vi "Relink Subroutine Test Exec.vi"(4 "Path Builder":refnum<class "IPath Builder.lvclass">, 6 "Persistence in":refnum<class "IPersist.lvclass">, 7 "Linked List ID":string, 8 "error in (no error)":errorcluster, 9 "Return":string, 10 "Subroutine Path":path, 11 "Linked List Ref":refnum<data-value>) -> (0 "error out":errorcluster, 1 "Return out":string, 3 "Linked List Ref out":refnum<data-value>)   [LabVIEW 2019, in "Test Executive.lvlib" / "Subroutine.lvclass"]
uses:
  <vilib>/gpm_packages/@cs/test-executive/Source/Test Executive/Subroutine/Subroutine.lvclass
  <vilib>/gpm_packages/@cs/linked-list/Source/Linked List/ILinkedList/ILinked List.lvclass
  <vilib>/gpm_packages/@cs/persistence/source/IPersist/IPersist.lvclass
  <vilib>/gpm_packages/@cs/test-executive/Source/Path Builder/IPath Builder/IPath Builder.lvclass
  <vilib>/gpm_packages/@cs/test-executive/Source/Test Executive/ITestExecutive/ITest Executive.lvclass
  <vilib>/gpm_packages/@cs/test-executive/Source/Test Executive/TestExecutive/Test Executive.lvclass
  C:/Program Files/National Instruments/LabVIEW 2019/vi.lib/gpm_packages/@cs/test-executive/Source/Test Executive/ITestExecutive/ITest Executive.lvclass
  99eec8f0-50ee-49f4-9012-2cedafc9663f.vi
  52bac3b5-23a8-4328-aead-fdf0a8238b8f.vi
  0dfa2f8a-f606-44bf-ad80-773e1d583f64.vi
  4a0ddc4e-31ac-45dd-9084-e524783595b4.vi
  7ffadc8e-1916-414d-bbdc-0be25d1b259b.vi
  448d75c9-5150-43a6-92ed-3c4cd4604ddf.vi
  49529079-acff-4e9f-a028-20bc5060d501.vi
  af76f34b-2ebe-473d-a8fe-d81e58e65588.vi
  ddc1e080-61ae-45a4-a330-8d8f04fba54d.vi
  <vilib>/Utility/error.llb/Error Cluster From Error Code.vi
  <vilib>/gpm_packages/@cs/test-executive/Source/Test Executive/TestExecutive Ref/TestExecutive Ref.lvclass
  <vilib>/gpm_packages/@cs/linked-list/Source/Linked List/Linked List Ref/Linked List Ref.lvclass
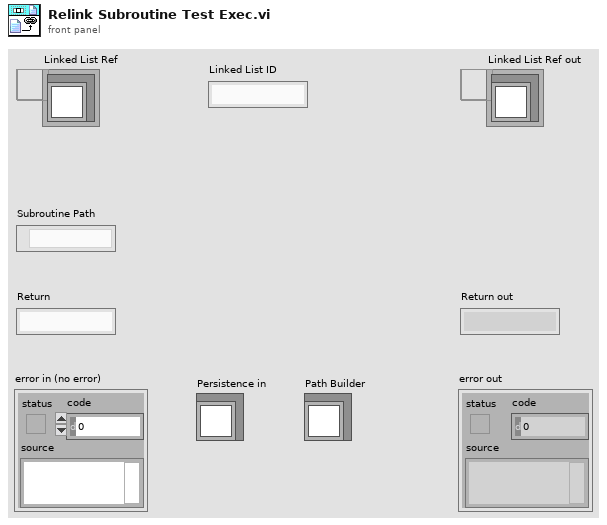
[diagram p1: front panel]
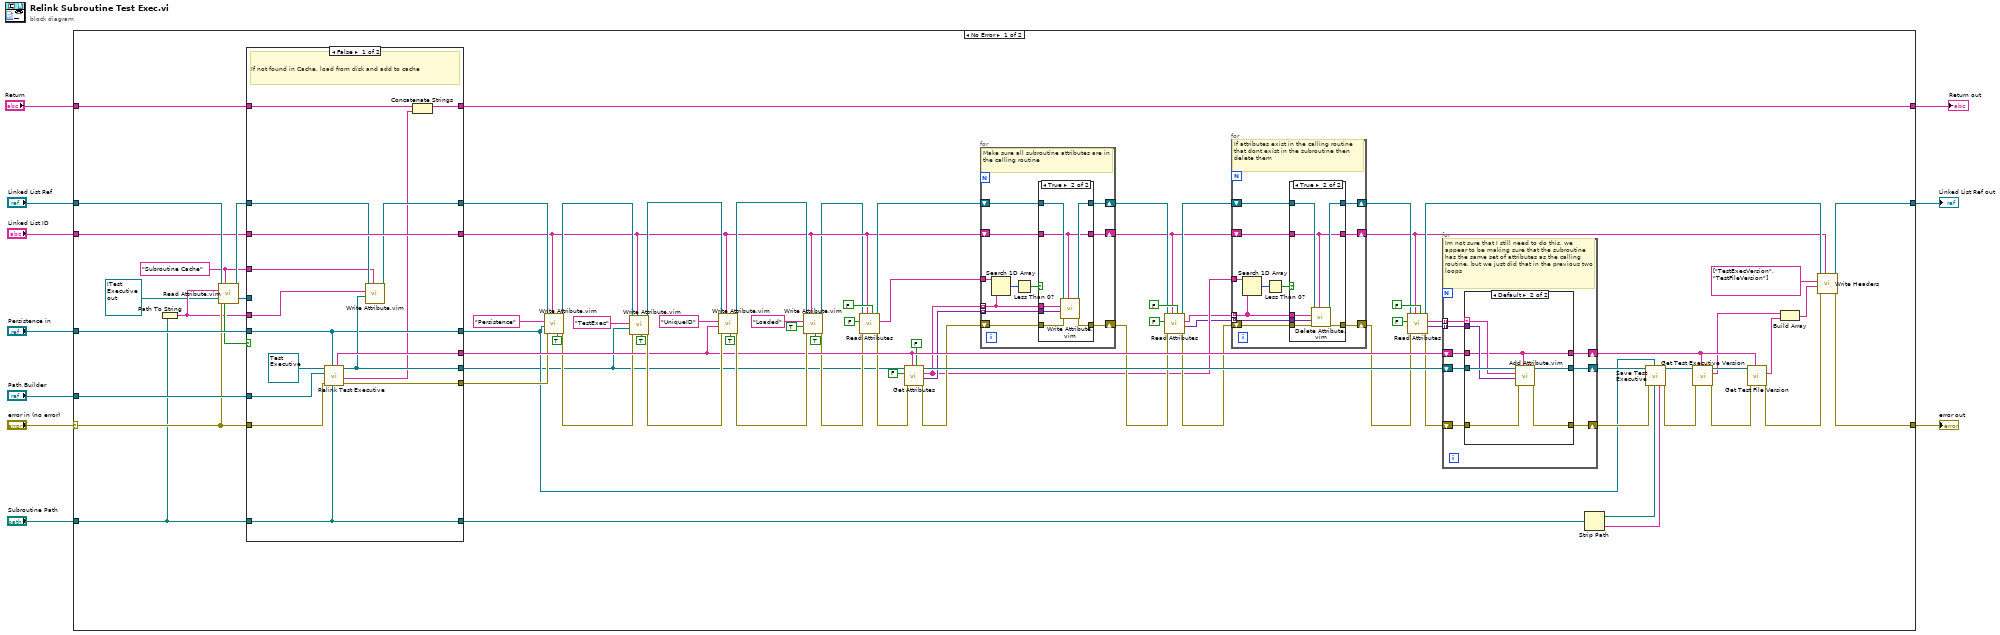
[diagram p0: block diagram]
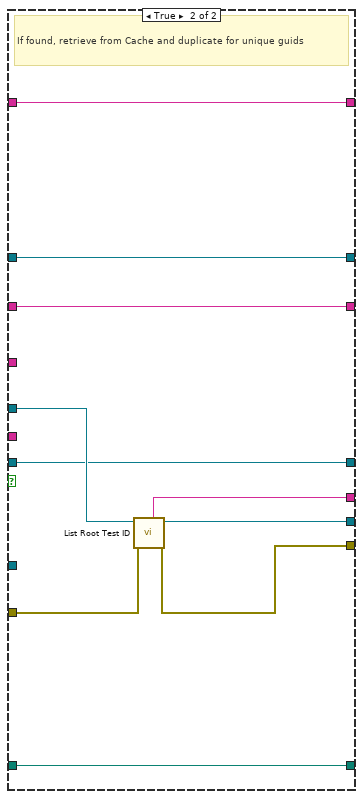
[diagram p2: hidden frame]
diagram:
  n1 = case shown="No Error" "error in (no error)" {
    selector: "error in (no error)" -> [w51 w181]
    tunnel: "Persistence in" -> [w84 _]
    tunnel: "Subroutine Path" -> [w50 _]
    tunnel: "Path Builder" -> [w83 _]
    tunnel: "Linked List Ref" -> [w52 w182]
    tunnel: "Linked List ID" -> [w47 _]
    tunnel: [w26 w182] -> w4
    tunnel: [w25 w181] -> w3
    tunnel: [w12 w180] -> w2
    tunnel: "Return" -> [w11 w180]
    frame No Error {
      w45 = "Subroutine Cache" ("Name")
      n2 = Path To String(path=w50) -> (string=w46:string)
      n3 = call "Read Attribute.vim"("Linked List Ref"=w52, "Linked List ID"=w45, "Attribute Name"=w46, "Type"=refnum<data-value> refnum ("Test Executive Ref out"), "error in (no error)"=w51) -> ("Linked List Ref out"=w48:refnum<data-value>, "Attribute"=w43:refnum<data-value>, "Found?"=w49:bool)  [unwired: 5 in, 3 out]
      n4 = case shown="False" w49 {
        tunnel: [w108 w116] -> w36
        tunnel: w84 -> [w99 w112]
        tunnel: w83 -> [w98 _]
        tunnel: [w100 w114] -> w13
        tunnel: [w101 w113] -> w77
        tunnel: w51 -> [w107 w117]
        tunnel: w50 -> [w97 w111]
        tunnel: [w104 w119] -> w39
        tunnel: w48 -> [w105 w119]
        tunnel: [w106 w118] -> w38
        tunnel: w47 -> [w106 w118]
        tunnel: w46 -> [w102 _]
        tunnel: w45 -> [w103 _]
        tunnel: w43 -> [_ w115]
        tunnel: [w99 w112] -> w33
        tunnel: [w97 w111] -> w32
        tunnel: [w95 w110] -> w12
        tunnel: w11 -> [w96 w110]
        frame False {
          # "If not found in Cache, load from disk and add to cache"
          n5 = call <vilib>:"Relink Test Executive.vi"("File"=w97, "Persistence in"=w99, "error in (no error)"=w107, "Path Builder"=w98, "Test Executive"=refnum<class "Test Executive.lvclass"> refnum ("Test Executive.lvlib:Test Executive.lvclass")) -> ("error out"=w108:errorcluster, "Return"=w94:string, "Test Executive Ref out"=w100:refnum<data-value>, "Root ID"=w101:string)  [unwired: 3 in]
          n6 = call "Write Attribute.vim"("Linked List ID"=w103, "Attribute"=w100, "Attribute Name"=w102, "Linked List Ref"=w105) -> ("Linked List Ref out"=w104:refnum<data-value>)  [unwired: 4 in, 3 out]
          n7 = Concatenate Strings(w96, w94) -> (w95:string)
        }
        frame True {
          # "If found, retrieve from Cache and duplicate for unique guids"
          n8 = call <vilib>:"List Root Test ID.vi"("error in (no error)"=w117, "Test Executive Ref"=w115) -> ("error out"=w116:errorcluster, "Test Executive Ref out"=w114:refnum<data-value>, "Root ID"=w113:string)  [unwired: 5 in, 2 out]
        }
      }
      n9 = call "Write Attribute.vim"("Private?"=TRUE, "Linked List ID"=w38, "error in (no error)"=w36, "Attribute"=w33, "Attribute Name"="Persistence", "Linked List Ref"=w39) -> ("error out"=w37:errorcluster, "Linked List Ref out"=w40:refnum<data-value>)  [unwired: 2 in, 2 out]
      n10 = call "Write Attribute.vim"("Private?"=TRUE, "Linked List ID"=w38, "error in (no error)"=w37, "Attribute"=w13, "Attribute Name"="TestExec", "Linked List Ref"=w40) -> ("error out"=w90:errorcluster, "Linked List Ref out"=w82:refnum<data-value>)  [unwired: 2 in, 2 out]
      n11 = call "Write Attribute.vim"("Private?"=TRUE, "Linked List ID"=w38, "error in (no error)"=w90, "Attribute"=w77, "Attribute Name"="UniqueID", "Linked List Ref"=w82) -> ("error out"=w86:errorcluster, "Linked List Ref out"=w81:refnum<data-value>)  [unwired: 2 in, 2 out]
      n12 = call "Write Attribute.vim"("Private?"=TRUE, "Linked List ID"=w38, "error in (no error)"=w86, "Attribute"=TRUE, "Attribute Name"="Loaded", "Linked List Ref"=w81) -> ("error out"=w28:errorcluster, "Linked List Ref out"=w29:refnum<data-value>)  [unwired: 2 in, 2 out]
      n13 = call <vilib>:"Read Attributes.vi"("Flatten Pointer?"=FALSE, "Linked List ID"=w38, "error in (no error)"=w28, "Include Private?"=FALSE, "Linked List Ref"=w29) -> ("error out"=w74:errorcluster, "Attribute Names out"=w73:string[], "Linked List Ref out"=w71:refnum<data-value>)  [unwired: 1 in, 3 out]
      n14 = call <vilib>:"Get Attributes.vi"("Flatten Pointer?"=FALSE, "Test ID"=w77, "error in (no error)"=w74, "Include Private?"=FALSE, "Test Executive Ref"=w13) -> ("error out"=w70:errorcluster, "Attributes"=w72:variant[], "Attribute Names out"=w62:string[], "Test Executive Ref out"=w78:refnum<data-value>)  [unwired: 1 in, 2 out]
      n15 = for {
        tunnel: w62 -> [w143] mode=indexing
        tunnel: w72 -> [w142] mode=indexing
        shift-right: [w148] -> w66
        shift-left: w71 -> [w149]
        tunnel: w73 -> [w150]
        shift-right: [w146] -> w67
        shift-left: w70 -> [w147]
        shift-right: [w141] -> w64
        shift-left: w38 -> [w145]
        # "Make sure all subroutine attributes are in the calling routine"
        n16 = Search 1D Array(1D array=w150, element=w143) -> (index of element=w151:i32)  [unwired: 1 in]
        n17 = Less Than 0?(x=w151) -> (x < 0?=w144:bool)
        n18 = case shown="True" w144 {
          tunnel: w149 -> [w154 w161]
          tunnel: [w154 w160] -> w148
          tunnel: w147 -> [w153 w159]
          tunnel: [w153 w158] -> w146
          tunnel: w145 -> [w152 w155]
          tunnel: w143 -> [_ w157]
          tunnel: w142 -> [_ w156]
          tunnel: [w152 w155] -> w141
          frame False {
          }
          frame True {
            n19 = call "Write Attribute.vim"("Linked List ID"=w155, "error in (no error)"=w159, "Attribute"=w156, "Attribute Name"=w157, "Linked List Ref"=w161) -> ("error out"=w158:errorcluster, "Linked List Ref out"=w160:refnum<data-value>)  [unwired: 3 in, 2 out]
          }
        }
      }
      n20 = call <vilib>:"Read Attributes.vi"("Flatten Pointer?"=FALSE, "Linked List ID"=w64, "error in (no error)"=w67, "Include Private?"=FALSE, "Linked List Ref"=w66) -> ("error out"=w63:errorcluster, "Attributes"=w60:variant[], "Attribute Names out"=w61:string[], "Linked List Ref out"=w65:refnum<data-value>)  [unwired: 1 in, 2 out]
      n21 = for {
        tunnel: w61 -> [w122] mode=indexing
        tunnel: w60 -> [w121] mode=indexing
        shift-right: [w127] -> w57
        shift-left: w65 -> [w128]
        tunnel: w62 -> [w129]
        shift-right: [w125] -> w56
        shift-left: w63 -> [w126]
        shift-right: [w120] -> w24
        shift-left: w64 -> [w124]
        # "If attributes exist in the calling routine that dont exist in the subroutine then delete them"
        n22 = Search 1D Array(1D array=w129, element=w122) -> (index of element=w130:i32)  [unwired: 1 in]
        n23 = Less Than 0?(x=w130) -> (x < 0?=w123:bool)
        n24 = case shown="True" w123 {
          tunnel: w128 -> [w133 w140]
          tunnel: [w133 w139] -> w127
          tunnel: w126 -> [w132 w137]
          tunnel: [w132 w136] -> w125
          tunnel: w124 -> [w131 w138]
          tunnel: w122 -> [_ w135]
          tunnel: w121 -> [_ w134]
          tunnel: [w131 w138] -> w120
          frame False {
          }
          frame True {
            n25 = call "Delete Attribute.vim"("Linked List ID"=w138, "error in (no error)"=w137, "Type"=w134, "Attribute Name"=w135, "Linked List Ref"=w140) -> ("error out"=w136:errorcluster, "Linked List Ref out"=w139:refnum<data-value>)  [unwired: 4 in, 1 out]
          }
        }
      }
      n26 = call <vilib>:"Read Attributes.vi"("Flatten Pointer?"=FALSE, "Linked List ID"=w24, "error in (no error)"=w56, "Include Private?"=FALSE, "Linked List Ref"=w57) -> ("error out"=w55:errorcluster, "Attributes"=w54:variant[], "Attribute Names out"=w53:string[], "Linked List Ref out"=w27:refnum<data-value>)  [unwired: 1 in, 2 out]
      n27 = for {
        shift-right: [w166] -> w34
        shift-left: w55 -> [w167]
        tunnel: w53 -> [w165] mode=indexing
        tunnel: w54 -> [w164] mode=indexing
        shift-right: [w163] -> w35
        shift-left: w78 -> [w169]
        shift-right: [w162] -> w17
        shift-left: w77 -> [w168]
        # "Im not sure that I still need to do this, we appear to be making sure that the subroutine has the same set of attributes as the calling routine, but we just did that in the previous two loops"
        n28 = case shown="Default" w165 {
          selector: w165 -> [_ w176]
          tunnel: w169 -> [w171 w179]
          tunnel: w168 -> [w170 w173]
          tunnel: w167 -> [w172 w178]
          tunnel: [w172 w177] -> w166
          tunnel: w164 -> [_ w175]
          tunnel: [w171 w174] -> w163
          tunnel: [w170 w173] -> w162
          frame "Restore Point" {
          }
          frame Default {
            n29 = call "Add Attribute.vim"("ID"=w173, "error in (no error)"=w178, "Attribute"=w175, "Attribute Name"=w176, "Test Executive Ref"=w179) -> ("error out"=w177:errorcluster, "Test Executive Ref out"=w174:refnum<data-value>)  [unwired: 3 in, 2 out]
          }
        }
      }
      n30 = Strip Path(path=w32) -> (stripped path=w31:path, name=w30:string)
      n31 = call <vilib>:"Save Test Executive.vi"("File Name"=w30, "Folder"=w31, "Persistence in"=w33, "error in (no error)"=w34, "Test Executive Ref"=w35) -> ("error out"=w20:errorcluster, "Test Executive Ref out"=w22:refnum<data-value>)  [unwired: 5 in]
      n32 = call <vilib>:"Get Test Executive Version.vi"("Unique ID"=w17, "error in (no error)"=w20, "Test Executive Ref"=w22) -> ("error out"=w18:errorcluster, "Test Executive Version"=w15:string, "Test Executive Ref out"=w21:refnum<data-value>)  [unwired: 5 in, 1 out]
      n33 = call <vilib>:"Get Test File Version.vi"("Unique ID"=w17, "error in (no error)"=w18, "Test Executive Ref"=w21) -> ("error out"=w19:errorcluster, "Test File Version"=w16:string)  [unwired: 5 in, 2 out]
      n34 = Build Array(w15, w16) -> (w14:string[])
      n35 = call <vilib>:"Write Headers.vi"("Linked List ID"=w24, "error in (no error)"=w19, "Header Values"=w14, "Header Names"=string[] ["TestExecVersion", "TestFileVersion"], "Linked List Ref"=w27) -> ("error out"=w25:errorcluster, "Linked List Ref out"=w26:refnum<data-value>)  [unwired: 5 in]
    }
    frame Error {
    }
  }
  "error out" <- w3
  "Linked List Ref out" <- w4
  "Return out" <- w2
